vi "CIF_CIPC_Tag Update Test Cases.vi"() -> (0 "error out":errorcluster, 2 "status":string, 3 "pass":bool)   [LabVIEW 2021]
uses:
  CIFChannels/Typedef/Direction.ctl
  Double/CIF_CIPC_Chn_Double.lvclass
  D:/dev/Packages/CIF_Channels_Core/src/CIFChannels/CIFChannels.lvclass
  U64/CIF_CIPC_Chn_U64.lvclass
  I64/CIF_CIPC_Chn_I64.lvclass
  a89bac37-e40b-4e23-8b15-caa5b580b70d.vi
  5767d73f-78c6-4091-81b3-8b4b134aad93.vi
  e629907d-3875-4979-a690-95404f934dc5.vi
  a89bac37-e40b-4e23-8b15-caa5b580b70d.vi/49b3dd2d-4579-4089-b72e-3f0875c862f2.vi
  <vilib>/CIF Foundation/CIF CIPC/SubVIs/Check Error.vi
  <vilib>/CIF Foundation/CIF CIPC/SubVIs/Get dll Path.vi
  <vilib>/CIF Foundation/CIF CIPC/SubVIs/Get Element Write Position.vi
  <vilib>/CIF Foundation/CIF CIPC/SubVIs/Notify Of New Write.vi
  <vilib>/CIF Foundation/CIF CIPC/SubVIs/Wait For N Elements Available.vi
  <vilib>/CIF Foundation/CIF CIPC/SubVIs/Get Element Read Position.vi
  <vilib>/CIF Foundation/CIF CIPC/SubVIs/Set Element Read Position.vi
  <vilib>/CIF Foundation/CIF CIPC/SubVIs/Get Element Description Variant.vi
  <vilib>/Utility/error.llb/Trim Whitespace.vi
  <vilib>/Utility/error.llb/Error Cluster From Error Code.vi
  <vilib>/CIF Foundation/CIF CIPC/SubVIs/Get Element Info Variant.vi
  CIFChannels/CIFChannels.lvclass
  <vilib>/CIF Foundation/CIF CIPC/CIF_NI_CIPC.lvlib
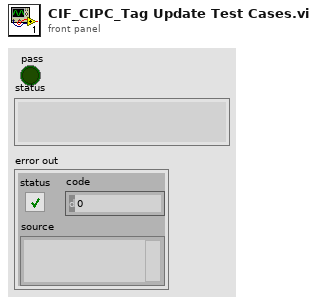
[diagram p1: front panel]
types:
  T1 = typedef "CIFChannels.lvclass/Direction.ctl" = enum16{"Publisher", "Subscriber"}
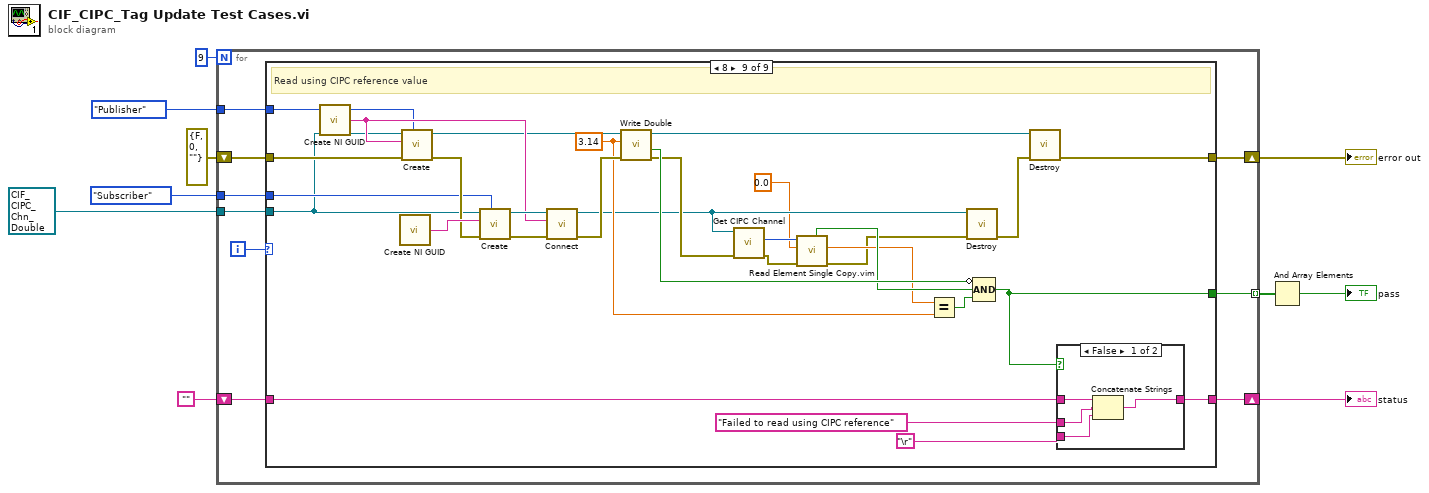
[diagram p0: block diagram]
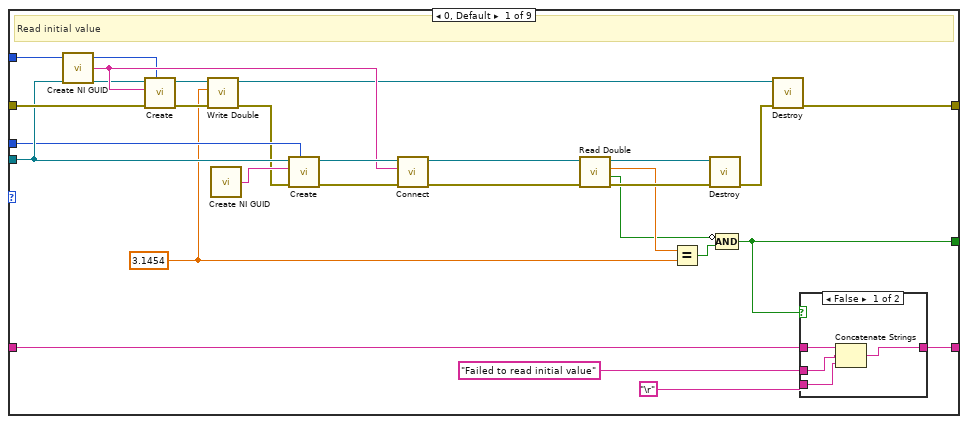
[diagram p2: hidden frame]
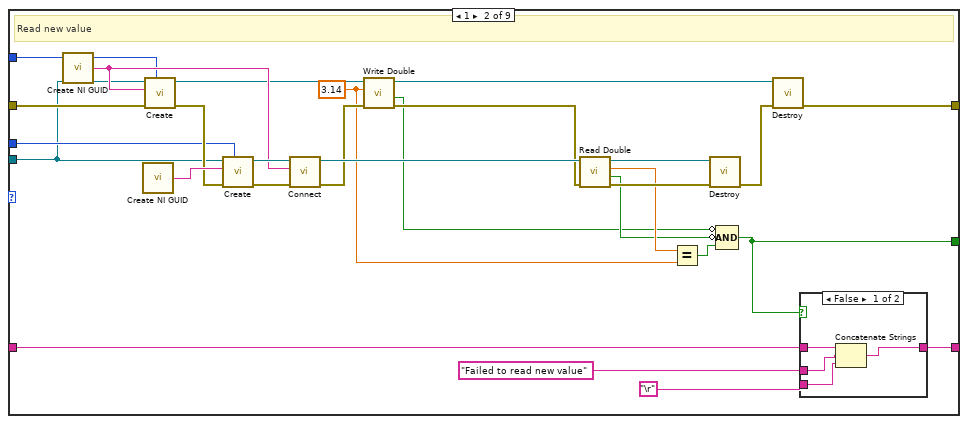
[diagram p4: hidden frame]
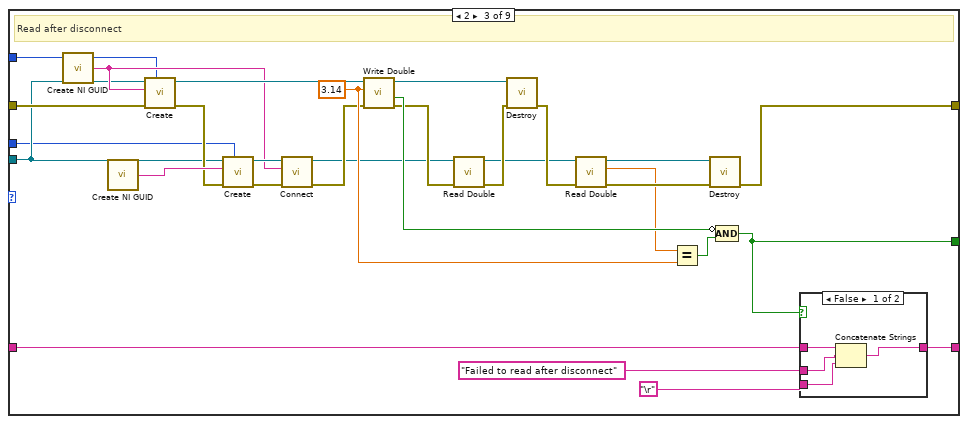
[diagram p6: hidden frame]
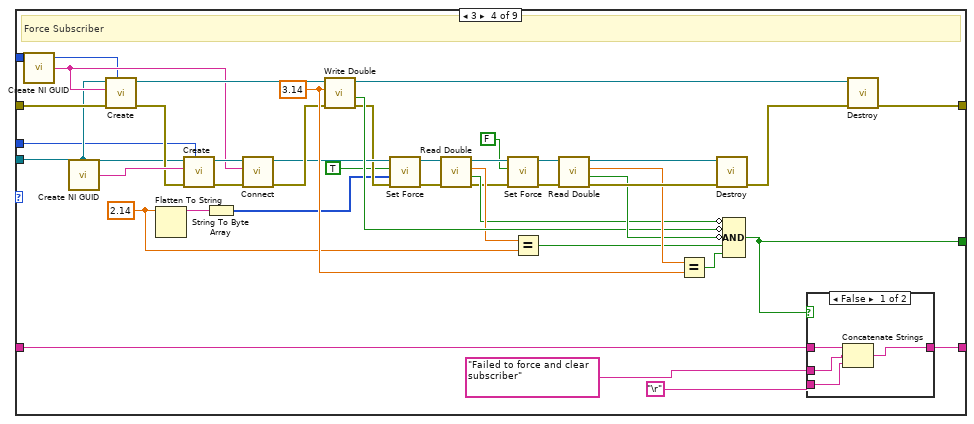
[diagram p8: hidden frame]
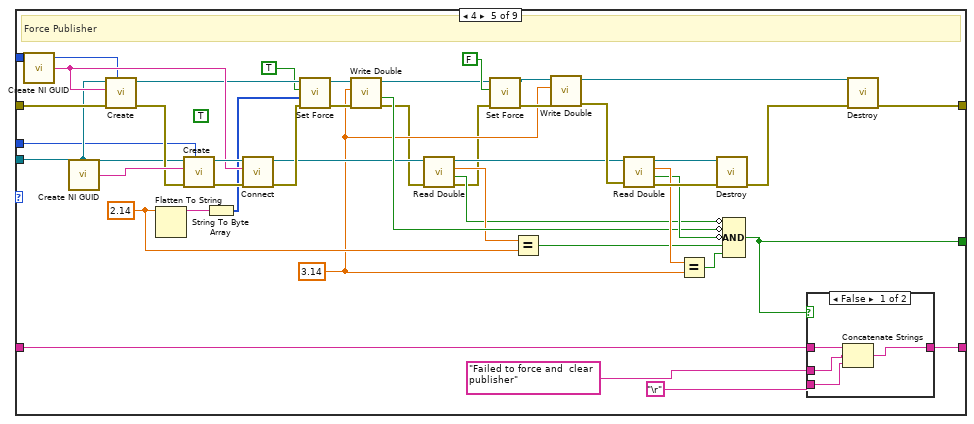
[diagram p10: hidden frame]
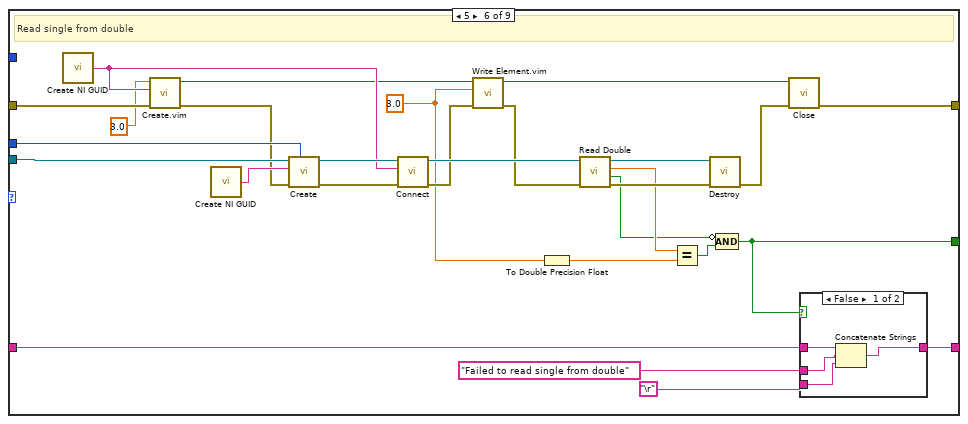
[diagram p12: hidden frame]
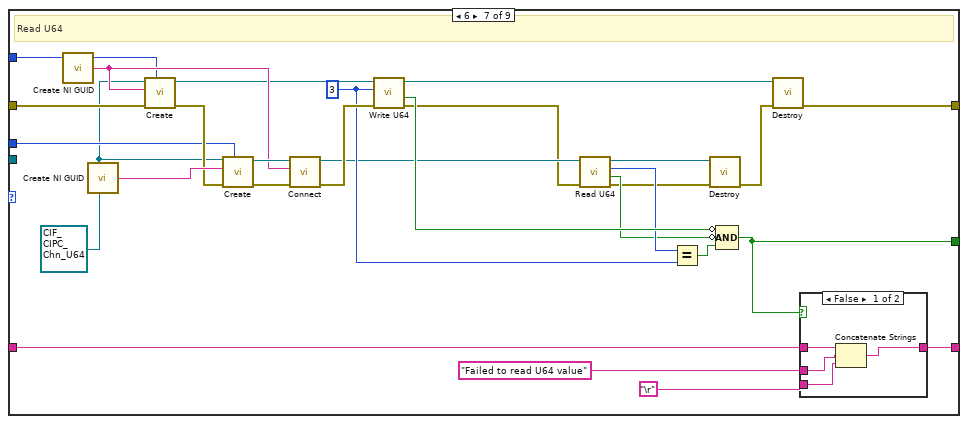
[diagram p14: hidden frame]
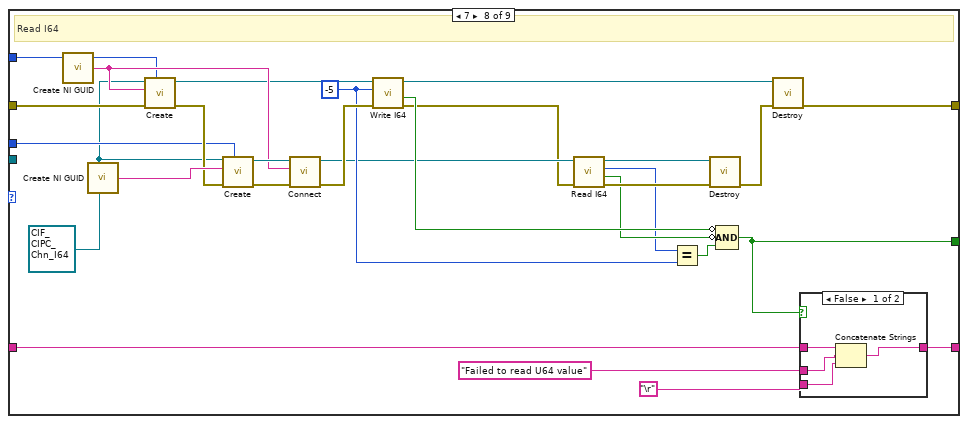
[diagram p16: hidden frame]
diagram:
  n1 = for {
    N: 9 -> [_]
    tunnel: [w19] -> w10 mode=indexing
    shift-right: [w17] -> w5
    shift-left: errorcluster {"status"=FALSE, "code"=0, "source"=""} ("error out") -> [w18]
    shift-right: [w14] -> w6
    shift-left: "" -> [w15]
    tunnel: refnum<class "CIF_CIPC_Chn_Double.lvclass"> refnum ("CIF_CIPC_Chn_Double.lvclass") -> [w13]
    tunnel: Direction."Publisher" ("Direction") -> [w12]
    tunnel: Direction."Subscriber" ("Direction") -> [w11]
    i -> [w16]
    n2 = case shown="8" w16 {
      tunnel: [w29 w62 w105 w150 w199 w230 w262 w295 w330] -> w19
      tunnel: w18 -> [w42 w75 w109 w156 w205 w222 w271 w304 w339]
      tunnel: [w32 w65 w98 w119 w182 w225 w264 w297 w332] -> w17
      tunnel: w15 -> [w46 w79 w113 w160 w209 w242 w275 w308 w343]
      tunnel: [w45 w78 w112 w159 w208 w241 w274 w307 w342] -> w14
      tunnel: w13 -> [w26 w52 w92 w140 w193 w228 _ _ w322]
      tunnel: w12 -> [w27 w54 w91 w139 w192 _ w261 w294 w324]
      tunnel: w11 -> [w25 w53 w90 w138 w191 w227 w260 w293 w323]
      frame 0, Default {
        w20 = 3.1454
        # "Read initial value"
        n3 = call <vilib>:"Create NI GUID.vi"() -> ("NI GUID"=w38:string)
        n4 = call-dynamic "Create.vi"("Direction"=w27, "error in (no error)"=w42, "Name"=w38, "CIFTag in"=w26) -> ("error out"=w23:errorcluster, "CIFTag out"=w24:refnum<class "CIF_CIPC_Chn_Double.lvclass">)  [unwired: 6 in]
        n5 = call-dynamic "Write Double.vi"("error in (no error)"=w23, "Data"=w20, "CIFTag in"=w24) -> ("error out"=w21:errorcluster, "CIFTag out"=w22:refnum<class "CIF_CIPC_Chn_Double.lvclass">)  [unwired: 6 in, 1 out]
        n6 = call <vilib>:"Create NI GUID.vi"() -> ("NI GUID"=w41:string)
        n7 = call-dynamic "Create.vi"("Direction"=w25, "error in (no error)"=w21, "Name"=w41, "CIFTag in"=w26) -> ("error out"=w39:errorcluster, "CIFTag out"=w40:refnum<class "CIF_CIPC_Chn_Double.lvclass">)  [unwired: 6 in]
        n8 = call-dynamic "Connect.vi"("error in (no error)"=w39, "Connection Name"=w38, "CIFTag in"=w40) -> ("error out"=w36:errorcluster, "CIFTag out"=w37:refnum<class "CIF_CIPC_Chn_Double.lvclass">)  [unwired: 7 in]
        n9 = call-dynamic "Read Double.vi"("error in (no error)"=w36, "CIFTag in"=w37) -> ("error out"=w34:errorcluster, "timed out?"=w28:bool, "Data"=w31:dbl, "CIFTag out"=w35:refnum<class "CIF_CIPC_Chn_Double.lvclass">)  [unwired: 6 in]
        n10 = Equal?(x=w31, y=w20) -> (x = y?=w30:bool)
        n11 = call-dynamic "Destroy.vi"("error in (no error)"=w34, "CIFTag in"=w35) -> ("error out"=w33:errorcluster)  [unwired: 8 in, 1 out]
        n12 = Compound Arithmetic op=AND(invert w28, w30) -> (w29:bool)
        n13 = call-dynamic "Destroy.vi"("error in (no error)"=w33, "CIFTag in"=w22) -> ("error out"=w32:errorcluster)  [unwired: 8 in, 1 out]
        n14 = case shown="False" w29 {
          tunnel: w46 -> [w50 w51]
          tunnel: [w47 w51] -> w45
          tunnel: "Failed to read initial value" -> [w49 _]
          tunnel: "\r" -> [w48 _]
          frame False {
            n15 = Concatenate Strings(w50, w49, w48) -> (w47:string)
          }
          frame True {
          }
        }
      }
      frame 1 {
        w55 = 3.14 ("Data")
        # "Read new value"
        n16 = call <vilib>:"Create NI GUID.vi"() -> ("NI GUID"=w70:string)
        n17 = call <vilib>:"Create NI GUID.vi"() -> ("NI GUID"=w74:string)
        n18 = call-dynamic "Create.vi"("Direction"=w54, "error in (no error)"=w75, "Name"=w70, "CIFTag in"=w52) -> ("error out"=w73:errorcluster, "CIFTag out"=w60:refnum<class "CIF_CIPC_Chn_Double.lvclass">)  [unwired: 6 in]
        n19 = call-dynamic "Create.vi"("Direction"=w53, "error in (no error)"=w73, "Name"=w74, "CIFTag in"=w52) -> ("error out"=w71:errorcluster, "CIFTag out"=w72:refnum<class "CIF_CIPC_Chn_Double.lvclass">)  [unwired: 6 in]
        n20 = call-dynamic "Connect.vi"("error in (no error)"=w71, "Connection Name"=w70, "CIFTag in"=w72) -> ("error out"=w59:errorcluster, "CIFTag out"=w69:refnum<class "CIF_CIPC_Chn_Double.lvclass">)  [unwired: 7 in]
        n21 = call-dynamic "Write Double.vi"("error in (no error)"=w59, "Data"=w55, "CIFTag in"=w60) -> ("error out"=w58:errorcluster, "timed out?"=w56:bool, "CIFTag out"=w57:refnum<class "CIF_CIPC_Chn_Double.lvclass">)  [unwired: 6 in]
        n22 = call-dynamic "Read Double.vi"("error in (no error)"=w58, "CIFTag in"=w69) -> ("error out"=w67:errorcluster, "timed out?"=w61:bool, "Data"=w64:dbl, "CIFTag out"=w68:refnum<class "CIF_CIPC_Chn_Double.lvclass">)  [unwired: 6 in]
        n23 = Equal?(x=w64, y=w55) -> (x = y?=w63:bool)
        n24 = call-dynamic "Destroy.vi"("error in (no error)"=w67, "CIFTag in"=w68) -> ("error out"=w66:errorcluster)  [unwired: 8 in, 1 out]
        n25 = Compound Arithmetic op=AND(invert w56, invert w61, w63) -> (w62:bool)
        n26 = call-dynamic "Destroy.vi"("error in (no error)"=w66, "CIFTag in"=w57) -> ("error out"=w65:errorcluster)  [unwired: 8 in, 1 out]
        n27 = case shown="False" w62 {
          tunnel: w79 -> [w83 w84]
          tunnel: [w80 w84] -> w78
          tunnel: "Failed to read new value" -> [w82 _]
          tunnel: "\r" -> [w81 _]
          frame False {
            n28 = Concatenate Strings(w83, w82, w81) -> (w80:string)
          }
          frame True {
          }
        }
      }
      frame 2 {
        w99 = 3.14 ("Data")
        # "Read after disconnect"
        n29 = call <vilib>:"Create NI GUID.vi"() -> ("NI GUID"=w93:string)
        n30 = call <vilib>:"Create NI GUID.vi"() -> ("NI GUID"=w108:string)
        n31 = call-dynamic "Create.vi"("Direction"=w91, "error in (no error)"=w109, "Name"=w93, "CIFTag in"=w92) -> ("error out"=w107:errorcluster, "CIFTag out"=w104:refnum<class "CIF_CIPC_Chn_Double.lvclass">)  [unwired: 6 in]
        n32 = call-dynamic "Create.vi"("Direction"=w90, "error in (no error)"=w107, "Name"=w108, "CIFTag in"=w92) -> ("error out"=w96:errorcluster, "CIFTag out"=w97:refnum<class "CIF_CIPC_Chn_Double.lvclass">)  [unwired: 6 in]
        n33 = call-dynamic "Connect.vi"("error in (no error)"=w96, "Connection Name"=w93, "CIFTag in"=w97) -> ("error out"=w95:errorcluster, "CIFTag out"=w94:refnum<class "CIF_CIPC_Chn_Double.lvclass">)  [unwired: 7 in]
        n34 = call-dynamic "Write Double.vi"("error in (no error)"=w95, "Data"=w99, "CIFTag in"=w104) -> ("error out"=w102:errorcluster, "timed out?"=w103:bool, "CIFTag out"=w101:refnum<class "CIF_CIPC_Chn_Double.lvclass">)  [unwired: 6 in]
        n35 = call-dynamic "Read Double.vi"("error in (no error)"=w102, "CIFTag in"=w94) -> ("error out"=w100:errorcluster, "CIFTag out"=w88:refnum<class "CIF_CIPC_Chn_Double.lvclass">)  [unwired: 6 in, 2 out]
        n36 = call-dynamic "Destroy.vi"("error in (no error)"=w100, "CIFTag in"=w101) -> ("error out"=w89:errorcluster)  [unwired: 8 in, 1 out]
        n37 = call-dynamic "Read Double.vi"("error in (no error)"=w89, "CIFTag in"=w88) -> ("error out"=w87:errorcluster, "Data"=w86:dbl, "CIFTag out"=w85:refnum<class "CIF_CIPC_Chn_Double.lvclass">)  [unwired: 6 in, 1 out]
        n38 = Equal?(x=w86, y=w99) -> (x = y?=w106:bool)
        n39 = call-dynamic "Destroy.vi"("error in (no error)"=w87, "CIFTag in"=w85) -> ("error out"=w98:errorcluster)  [unwired: 8 in, 1 out]
        n40 = Compound Arithmetic op=AND(invert w103, w106) -> (w105:bool)
        n41 = case shown="False" w105 {
          tunnel: w113 -> [w117 w118]
          tunnel: [w114 w118] -> w112
          tunnel: "Failed to read after disconnect" -> [w116 _]
          tunnel: "\r" -> [w115 _]
          frame False {
            n42 = Concatenate Strings(w117, w116, w115) -> (w114:string)
          }
          frame True {
          }
        }
      }
      frame 3 {
        w129 = 2.14 ("Data")
        w145 = 3.14 ("Data")
        # "Force Subscriber"
        n43 = call <vilib>:"Create NI GUID.vi"() -> ("NI GUID"=w141:string)
        n44 = call <vilib>:"Create NI GUID.vi"() -> ("NI GUID"=w155:string)
        n45 = call-dynamic "Create.vi"("Direction"=w139, "error in (no error)"=w156, "Name"=w141, "CIFTag in"=w140) -> ("error out"=w154:errorcluster, "CIFTag out"=w148:refnum<class "CIF_CIPC_Chn_Double.lvclass">)  [unwired: 6 in]
        n46 = Flatten To String(anything=w129) -> (data string=w135:string)  [unwired: 3 in, 2 out]
        n47 = call-dynamic "Create.vi"("Direction"=w138, "error in (no error)"=w154, "Name"=w155, "CIFTag in"=w140) -> ("error out"=w143:errorcluster, "CIFTag out"=w144:refnum<class "CIF_CIPC_Chn_Double.lvclass">)  [unwired: 6 in]
        n48 = String To Byte Array(string=w135) -> (unsigned byte array=w134:u8[])
        n49 = call-dynamic "Connect.vi"("error in (no error)"=w143, "Connection Name"=w141, "CIFTag in"=w144) -> ("error out"=w142:errorcluster, "CIFTag out"=w137:refnum<class "CIF_CIPC_Chn_Double.lvclass">)  [unwired: 7 in]
        n50 = call-dynamic "Write Double.vi"("error in (no error)"=w142, "Data"=w145, "CIFTag in"=w148) -> ("error out"=w136:errorcluster, "timed out?"=w147:bool, "CIFTag out"=w146:refnum<class "CIF_CIPC_Chn_Double.lvclass">)  [unwired: 6 in]
        n51 = call "Set Force.vi"("error in (no error)"=w136, "Force Data"=w134, "Force Active"=TRUE, "CIFChannels in"=w137) -> ("error out"=w131:errorcluster, "CIFChannels out"=w132:refnum<class "CIF_CIPC_Chn_Double.lvclass">)  [unwired: 6 in]
        n52 = call-dynamic "Read Double.vi"("error in (no error)"=w131, "CIFTag in"=w132) -> ("error out"=w124:errorcluster, "timed out?"=w128:bool, "Data"=w130:dbl, "CIFTag out"=w125:refnum<class "CIF_CIPC_Chn_Double.lvclass">)  [unwired: 6 in]
        n53 = call "Set Force.vi"("error in (no error)"=w124, "Force Active"=FALSE, "CIFChannels in"=w125) -> ("error out"=w123:errorcluster, "CIFChannels out"=w122:refnum<class "CIF_CIPC_Chn_Double.lvclass">)  [unwired: 7 in]
        n54 = Equal?(x=w130, y=w129) -> (x = y?=w126:bool)
        n55 = call-dynamic "Read Double.vi"("error in (no error)"=w123, "CIFTag in"=w122) -> ("error out"=w152:errorcluster, "timed out?"=w149:bool, "Data"=w151:dbl, "CIFTag out"=w153:refnum<class "CIF_CIPC_Chn_Double.lvclass">)  [unwired: 6 in]
        n56 = Equal?(x=w151, y=w145) -> (x = y?=w127:bool)
        n57 = call-dynamic "Destroy.vi"("error in (no error)"=w152, "CIFTag in"=w153) -> ("error out"=w120:errorcluster)  [unwired: 8 in, 1 out]
        n58 = Compound Arithmetic op=AND(invert w128, invert w147, invert w149, w126, w127) -> (w150:bool)
        n59 = case shown="False" w150 {
          tunnel: w160 -> [w164 w165]
          tunnel: [w161 w165] -> w159
          tunnel: "Failed to force and clear subscriber" -> [w163 _]
          tunnel: "\r" -> [w162 _]
          frame False {
            n60 = Concatenate Strings(w164, w163, w162) -> (w161:string)
          }
          frame True {
          }
        }
        n61 = call-dynamic "Destroy.vi"("error in (no error)"=w120, "CIFTag in"=w146) -> ("error out"=w119:errorcluster)  [unwired: 8 in, 1 out]
      }
      frame 4 {
        (unwired) TRUE ("Force Active")
        w188 = 2.14 ("Data")
        w171 = 3.14 ("Data")
        # "Force Publisher"
        n62 = call <vilib>:"Create NI GUID.vi"() -> ("NI GUID"=w194:string)
        n63 = call <vilib>:"Create NI GUID.vi"() -> ("NI GUID"=w204:string)
        n64 = call-dynamic "Create.vi"("Direction"=w192, "error in (no error)"=w205, "Name"=w194, "CIFTag in"=w193) -> ("error out"=w203:errorcluster, "CIFTag out"=w181:refnum<class "CIF_CIPC_Chn_Double.lvclass">)  [unwired: 6 in]
        n65 = Flatten To String(anything=w188) -> (data string=w190:string)  [unwired: 3 in, 2 out]
        n66 = call-dynamic "Create.vi"("Direction"=w191, "error in (no error)"=w203, "Name"=w204, "CIFTag in"=w193) -> ("error out"=w195:errorcluster, "CIFTag out"=w196:refnum<class "CIF_CIPC_Chn_Double.lvclass">)  [unwired: 6 in]
        n67 = String To Byte Array(string=w190) -> (unsigned byte array=w180:u8[])
        n68 = call-dynamic "Connect.vi"("error in (no error)"=w195, "Connection Name"=w194, "CIFTag in"=w196) -> ("error out"=w177:errorcluster, "CIFTag out"=w175:refnum<class "CIF_CIPC_Chn_Double.lvclass">)  [unwired: 7 in]
        n69 = call "Set Force.vi"("error in (no error)"=w177, "Force Data"=w180, "Force Active"=TRUE, "CIFChannels in"=w181) -> ("error out"=w178:errorcluster, "CIFChannels out"=w179:refnum<class "CIF_CIPC_Chn_Double.lvclass">)  [unwired: 6 in]
        n70 = call-dynamic "Write Double.vi"("error in (no error)"=w178, "Data"=w171, "CIFTag in"=w179) -> ("error out"=w167:errorcluster, "timed out?"=w197:bool, "CIFTag out"=w174:refnum<class "CIF_CIPC_Chn_Double.lvclass">)  [unwired: 6 in]
        n71 = call-dynamic "Read Double.vi"("error in (no error)"=w167, "CIFTag in"=w175) -> ("error out"=w166:errorcluster, "timed out?"=w187:bool, "Data"=w189:dbl, "CIFTag out"=w168:refnum<class "CIF_CIPC_Chn_Double.lvclass">)  [unwired: 6 in]
        n72 = call "Set Force.vi"("error in (no error)"=w166, "Force Active"=FALSE, "CIFChannels in"=w174) -> ("error out"=w173:errorcluster, "CIFChannels out"=w172:refnum<class "CIF_CIPC_Chn_Double.lvclass">)  [unwired: 7 in]
        n73 = Equal?(x=w189, y=w188) -> (x = y?=w185:bool)
        n74 = call-dynamic "Write Double.vi"("error in (no error)"=w173, "Data"=w171, "CIFTag in"=w172) -> ("error out"=w170:errorcluster, "CIFTag out"=w169:refnum<class "CIF_CIPC_Chn_Double.lvclass">)  [unwired: 6 in, 1 out]
        n75 = call-dynamic "Read Double.vi"("error in (no error)"=w170, "CIFTag in"=w168) -> ("error out"=w201:errorcluster, "timed out?"=w198:bool, "Data"=w200:dbl, "CIFTag out"=w202:refnum<class "CIF_CIPC_Chn_Double.lvclass">)  [unwired: 6 in]
        n76 = Equal?(x=w200, y=w171) -> (x = y?=w186:bool)
        n77 = call-dynamic "Destroy.vi"("error in (no error)"=w201, "CIFTag in"=w202) -> ("error out"=w183:errorcluster)  [unwired: 8 in, 1 out]
        n78 = Compound Arithmetic op=AND(invert w187, invert w197, invert w198, w185, w186) -> (w199:bool)
        n79 = case shown="False" w199 {
          tunnel: w209 -> [w213 w214]
          tunnel: [w210 w214] -> w208
          tunnel: "Failed to force and  clear publisher" -> [w212 _]
          tunnel: "\r" -> [w211 _]
          frame False {
            n80 = Concatenate Strings(w213, w212, w211) -> (w210:string)
          }
          frame True {
          }
        }
        n81 = call-dynamic "Destroy.vi"("error in (no error)"=w183, "CIFTag in"=w169) -> ("error out"=w182:errorcluster)  [unwired: 8 in, 1 out]
      }
      frame 5 {
        w217 = sgl 3.0
        # "Read single from double"
        n82 = call <vilib>:"Create NI GUID.vi"() -> ("NI GUID"=w221:string)
        n83 = call "Create.vim"("error in (no error)"=w222, "Name in"=w221, "Data Type"=sgl 3.0) -> ("error out"=w219:errorcluster, "CIPC Reference"=w218:u64)  [unwired: 5 in, 2 out]
        n84 = call <vilib>:"Create NI GUID.vi"() -> ("NI GUID"=w238:string)
        n85 = call-dynamic "Create.vi"("Direction"=w227, "error in (no error)"=w219, "Name"=w238, "CIFTag in"=w228) -> ("error out"=w236:errorcluster, "CIFTag out"=w237:refnum<class "CIF_CIPC_Chn_Double.lvclass">)  [unwired: 6 in]
        n86 = call-dynamic "Connect.vi"("error in (no error)"=w236, "Connection Name"=w221, "CIFTag in"=w237) -> ("error out"=w224:errorcluster, "CIFTag out"=w235:refnum<class "CIF_CIPC_Chn_Double.lvclass">)  [unwired: 7 in]
        n87 = call "Write Element.vim"("error in (no error)"=w224, "Data in"=w217, "CIPC Reference in"=w218) -> ("error out"=w223:errorcluster, "CIPC Reference out"=w216:u64)  [unwired: 5 in, 2 out]
        n88 = To Double Precision Float(number=w217) -> (double precision float=w215:dbl)
        n89 = call-dynamic "Read Double.vi"("error in (no error)"=w223, "CIFTag in"=w235) -> ("error out"=w233:errorcluster, "timed out?"=w229:bool, "Data"=w232:dbl, "CIFTag out"=w234:refnum<class "CIF_CIPC_Chn_Double.lvclass">)  [unwired: 6 in]
        n90 = Equal?(x=w232, y=w215) -> (x = y?=w231:bool)
        n91 = call-dynamic "Destroy.vi"("error in (no error)"=w233, "CIFTag in"=w234) -> ("error out"=w226:errorcluster)  [unwired: 8 in, 1 out]
        n92 = Compound Arithmetic op=AND(invert w229, w231) -> (w230:bool)
        n93 = call <vilib>:"Close.vi"("error in (no error)"=w226, "CIPC Reference"=w216) -> ("error out"=w225:errorcluster)  [unwired: 9 in]
        n94 = case shown="False" w230 {
          tunnel: w242 -> [w246 w247]
          tunnel: [w243 w247] -> w241
          tunnel: "Failed to read single from double" -> [w245 _]
          tunnel: "\r" -> [w244 _]
          frame False {
            n95 = Concatenate Strings(w246, w245, w244) -> (w243:string)
          }
          frame True {
          }
        }
      }
      frame 6 {
        w259 = refnum<class "CIF_CIPC_Chn_U64.lvclass"> refnum ("CIF_CIPC_Chn_U64.lvclass")
        w254 = u64 3 ("Data")
        # "Read U64"
        n96 = call <vilib>:"Create NI GUID.vi"() -> ("NI GUID"=w266:string)
        n97 = call <vilib>:"Create NI GUID.vi"() -> ("NI GUID"=w270:string)
        n98 = call-dynamic "Create.vi"("Direction"=w261, "error in (no error)"=w271, "Name"=w266, "CIFTag in"=w259) -> ("error out"=w269:errorcluster, "CIFTag out"=w257:refnum<class "CIF_CIPC_Chn_U64.lvclass">)  [unwired: 6 in]
        n99 = call-dynamic "Create.vi"("Direction"=w260, "error in (no error)"=w269, "Name"=w270, "CIFTag in"=w259) -> ("error out"=w267:errorcluster, "CIFTag out"=w268:refnum<class "CIF_CIPC_Chn_U64.lvclass">)  [unwired: 6 in]
        n100 = call-dynamic "Connect.vi"("error in (no error)"=w267, "Connection Name"=w266, "CIFTag in"=w268) -> ("error out"=w258:errorcluster, "CIFTag out"=w253:refnum<class "CIF_CIPC_Chn_U64.lvclass">)  [unwired: 7 in]
        n101 = call-dynamic "Write U64.vi"("error in (no error)"=w258, "Data"=w254, "CIFTag in"=w257) -> ("error out"=w252:errorcluster, "timed out?"=w255:bool, "CIFTag out"=w256:refnum<class "CIF_CIPC_Chn_U64.lvclass">)  [unwired: 6 in]
        n102 = call-dynamic "Read U64.vi"("error in (no error)"=w252, "CIFTag in"=w253) -> ("error out"=w248:errorcluster, "timed out?"=w249:bool, "Data"=w250:u64, "CIFTag out"=w251:refnum<class "CIF_CIPC_Chn_U64.lvclass">)  [unwired: 6 in]
        n103 = Equal?(x=w250, y=w254) -> (x = y?=w263:bool)
        n104 = call-dynamic "Destroy.vi"("error in (no error)"=w248, "CIFTag in"=w251) -> ("error out"=w265:errorcluster)  [unwired: 8 in, 1 out]
        n105 = Compound Arithmetic op=AND(invert w255, invert w249, w263) -> (w262:bool)
        n106 = call-dynamic "Destroy.vi"("error in (no error)"=w265, "CIFTag in"=w256) -> ("error out"=w264:errorcluster)  [unwired: 8 in, 1 out]
        n107 = case shown="False" w262 {
          tunnel: w275 -> [w279 w280]
          tunnel: [w276 w280] -> w274
          tunnel: "Failed to read U64 value" -> [w278 _]
          tunnel: "\r" -> [w277 _]
          frame False {
            n108 = Concatenate Strings(w279, w278, w277) -> (w276:string)
          }
          frame True {
          }
        }
      }
      frame 7 {
        w281 = refnum<class "CIF_CIPC_Chn_I64.lvclass"> refnum ("CIF_CIPC_Chn_I64.lvclass")
        w290 = i64 -5 ("Data")
        # "Read I64"
        n109 = call <vilib>:"Create NI GUID.vi"() -> ("NI GUID"=w299:string)
        n110 = call <vilib>:"Create NI GUID.vi"() -> ("NI GUID"=w303:string)
        n111 = call-dynamic "Create.vi"("Direction"=w294, "error in (no error)"=w304, "Name"=w299, "CIFTag in"=w281) -> ("error out"=w302:errorcluster, "CIFTag out"=w292:refnum<class "CIF_CIPC_Chn_I64.lvclass">)  [unwired: 6 in]
        n112 = call-dynamic "Create.vi"("Direction"=w293, "error in (no error)"=w302, "Name"=w303, "CIFTag in"=w281) -> ("error out"=w300:errorcluster, "CIFTag out"=w301:refnum<class "CIF_CIPC_Chn_I64.lvclass">)  [unwired: 6 in]
        n113 = call-dynamic "Connect.vi"("error in (no error)"=w300, "Connection Name"=w299, "CIFTag in"=w301) -> ("error out"=w291:errorcluster, "CIFTag out"=w287:refnum<class "CIF_CIPC_Chn_I64.lvclass">)  [unwired: 7 in]
        n114 = call-dynamic "Write I64.vi"("error in (no error)"=w291, "Data"=w290, "CIFTag in"=w292) -> ("error out"=w286:errorcluster, "timed out?"=w288:bool, "CIFTag out"=w289:refnum<class "CIF_CIPC_Chn_I64.lvclass">)  [unwired: 6 in]
        n115 = call-dynamic "Read I64.vi"("error in (no error)"=w286, "CIFTag in"=w287) -> ("error out"=w285:errorcluster, "timed out?"=w284:bool, "Data"=w283:i64, "CIFTag out"=w282:refnum<class "CIF_CIPC_Chn_I64.lvclass">)  [unwired: 6 in]
        n116 = Equal?(x=w283, y=w290) -> (x = y?=w296:bool)
        n117 = call-dynamic "Destroy.vi"("error in (no error)"=w285, "CIFTag in"=w282) -> ("error out"=w298:errorcluster)  [unwired: 8 in, 1 out]
        n118 = Compound Arithmetic op=AND(invert w288, invert w284, w296) -> (w295:bool)
        n119 = call-dynamic "Destroy.vi"("error in (no error)"=w298, "CIFTag in"=w289) -> ("error out"=w297:errorcluster)  [unwired: 8 in, 1 out]
        n120 = case shown="False" w295 {
          tunnel: w308 -> [w312 w313]
          tunnel: [w309 w313] -> w307
          tunnel: "Failed to read U64 value" -> [w311 _]
          tunnel: "\r" -> [w310 _]
          frame False {
            n121 = Concatenate Strings(w312, w311, w310) -> (w309:string)
          }
          frame True {
          }
        }
      }
      frame 8 {
        w325 = 3.14 ("Data")
        # "Read using CIPC reference value"
        n122 = call <vilib>:"Create NI GUID.vi"() -> ("NI GUID"=w334:string)
        n123 = call <vilib>:"Create NI GUID.vi"() -> ("NI GUID"=w338:string)
        n124 = call-dynamic "Create.vi"("Direction"=w324, "error in (no error)"=w339, "Name"=w334, "CIFTag in"=w322) -> ("error out"=w337:errorcluster, "CIFTag out"=w329:refnum<class "CIF_CIPC_Chn_Double.lvclass">)  [unwired: 6 in]
        n125 = call-dynamic "Create.vi"("Direction"=w323, "error in (no error)"=w337, "Name"=w338, "CIFTag in"=w322) -> ("error out"=w335:errorcluster, "CIFTag out"=w336:refnum<class "CIF_CIPC_Chn_Double.lvclass">)  [unwired: 6 in]
        n126 = call-dynamic "Connect.vi"("error in (no error)"=w335, "Connection Name"=w334, "CIFTag in"=w336) -> ("error out"=w328:errorcluster, "CIFTag out"=w320:refnum<class "CIF_CIPC_Chn_Double.lvclass">)  [unwired: 7 in]
        n127 = call-dynamic "Write Double.vi"("error in (no error)"=w328, "Data"=w325, "CIFTag in"=w329) -> ("error out"=w321:errorcluster, "timed out?"=w326:bool, "CIFTag out"=w327:refnum<class "CIF_CIPC_Chn_Double.lvclass">)  [unwired: 6 in]
        n128 = call-dynamic "Get CIPC Channel.vi"("error in (no error)"=w321, "CIF_CIPC_Chn in"=w320) -> ("error out"=w314:errorcluster, "CIPC Channel"=w319:u64)  [unwired: 7 in, 1 out]
        n129 = call "Read Element Single Copy.vim"("error in (no error)"=w314, "Data in"=0.0 ("Data"), "CIPC Reference in"=w319) -> ("error out"=w315:errorcluster, "Data out"=w316:dbl, "Success"=w317:bool)  [unwired: 4 in, 2 out]
        n130 = Equal?(x=w316, y=w325) -> (x = y?=w331:bool)
        n131 = call-dynamic "Destroy.vi"("error in (no error)"=w315, "CIFTag in"=w320) -> ("error out"=w333:errorcluster)  [unwired: 8 in, 1 out]
        n132 = Compound Arithmetic op=AND(invert w326, w317, w331) -> (w330:bool)
        n133 = call-dynamic "Destroy.vi"("error in (no error)"=w333, "CIFTag in"=w327) -> ("error out"=w332:errorcluster)  [unwired: 8 in, 1 out]
        n134 = case shown="False" w330 {
          tunnel: w343 -> [w347 w348]
          tunnel: [w344 w348] -> w342
          tunnel: "Failed to read using CIPC reference" -> [w346 _]
          tunnel: "\r" -> [w345 _]
          frame False {
            n135 = Concatenate Strings(w347, w346, w345) -> (w344:string)
          }
          frame True {
          }
        }
      }
    }
  }
  "error out" <- w5
  "status" <- w6
  n136 = And Array Elements(Boolean array=w10) -> (logical AND=→"pass":bool)
